vi "Send and Forget Data Response.vi"(8 "error in (no error)":errorcluster, 11 "Response Core in":refnum<class "Response Core.lvclass">) -> (0 "error out":errorcluster, 3 "Data":refnum<class "Data.lvclass">)   [LabVIEW 2020, in "Publisher.lvlib" / "Response Core.lvclass"]
doc: "Data generated from the response core when a message is sent as 'Send and Forget'.\n\nThe default implementation returns an empty Data class."
uses:
  Response Core.lvclass
  PPL/HDH.Data.Generic.lvlibp/Data.lvclass
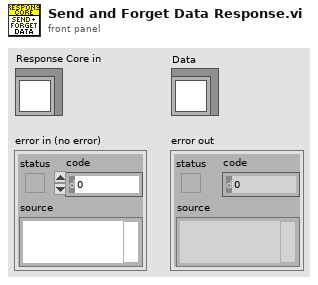
[diagram p1: front panel]
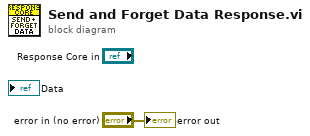
[diagram p0: block diagram]
diagram:
  "error out" <- "error in (no error)"
